vi "TB-Update Spectrum Average.vi"(5 "mic signal":dbl[](array[numeric]), 7 "state in":T1) -> (4 "RMS":dbl, 6 "+Freq. Mag of FFT (dB rms) out":dbl[](array[numeric]), 8 "state out":T1)   [LabVIEW 2020]
uses:
  Typedefs/TB-Runtime state.ctl
  <vilib>/sound2/lvsound2.llb/Sound File Refnum.ctl
  Typedefs/TB-Setup Log.ctl
  <vilib>/Analysis/baseanly.llb/Mean.vi
  <vilib>/Analysis/baseanly.llb/Mean (DBL).vi
  epl-vi-lib/Utility VIs/Math VIs/FFT x(t) to dB,Degrees (1D).vi
  epl-vi-lib/Utility VIs/Math VIs/dB to Linear (1D).vi
  epl-vi-lib/Utility VIs/Math VIs/Linear to dB (scalar).vi
  epl-vi-lib/Utility VIs/Math VIs/Linear to dB (array).vi
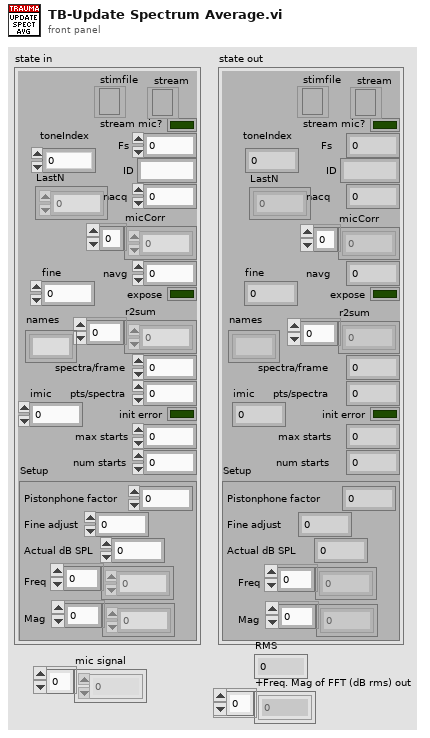
[diagram p1: front panel]
types:
  T1 = typedef "TB-Runtime state.ctl" = cluster{"stimfile":T2, "stream mic?":bool, "Fs":dbl, "ID":string, "micCorr":dbl[], "navg":i32, "r2sum":dbl[], "expose":bool, "spectra/frame":i32, "pts/spectra":i32, "nacq":i32, "init error":bool, "max starts":i32, "num starts":i32, "Setup":T3, "toneIndex":i32, "LastN":dbl[], "fine":dbl, "imic":i32, "stream":refnum<file>, "names":string[]}
  T2 = typedef "Sound File Refnum.ctl" = refnum<file>
  T3 = typedef "TB-Setup Log.ctl" = cluster{"Pistonphone factor":dbl, "Fine adjust":dbl, "Actual dB SPL":dbl, "Freq":dbl[], "Mag":dbl[]}
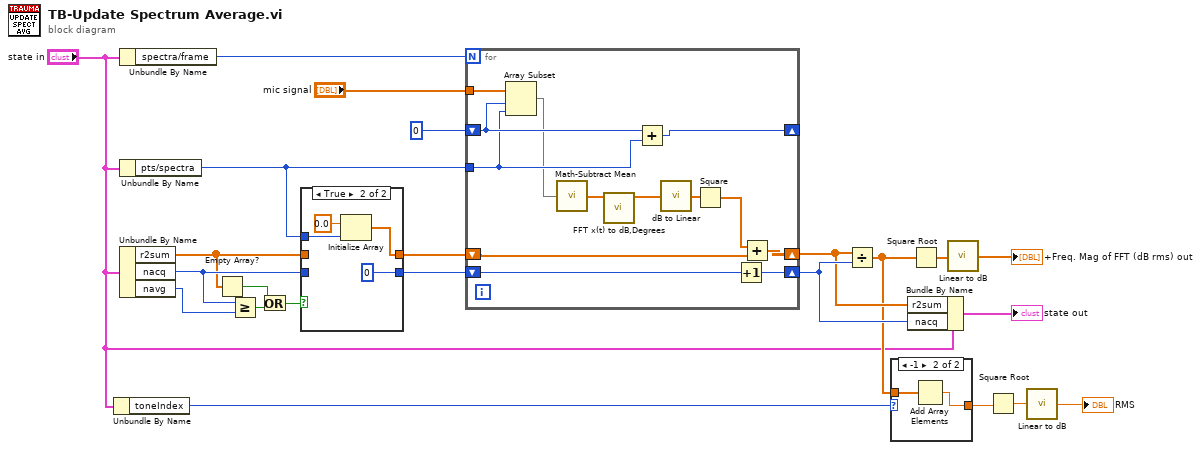
[diagram p0: block diagram]
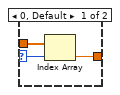
[diagram p3: hidden frame]
diagram:
  n1 = Unbundle By Name("state in") -> ("toneIndex"=w3:i32)
  n2 = Unbundle By Name("state in") -> ("spectra/frame"=w11:i32)
  n3 = Unbundle By Name("state in") -> ("pts/spectra"=w12:i32)
  n4 = Unbundle By Name("state in") -> ("r2sum"=w15:dbl[], "nacq"=w20:i32, "navg"=w10:i32)
  n5 = Empty Array?(array=w15) -> (empty?=w22:bool)
  n6 = Greater Or Equal?(x=w20, y=w10) -> (x >= y?=w23:bool)
  n7 = Or(x=w22, y=w23) -> (x .or. y?=w21:bool)
  n8 = case shown="True" w21 {
    tunnel: w15 -> [w25 _]
    tunnel: [w25 w26] -> w13
    tunnel: w20 -> [w24 _]
    tunnel: [w24 0] -> w14
    tunnel: w12 -> [_ w28]
    frame False {
    }
    frame True {
      n9 = Initialize Array(0.0 ("element"), w28) -> (w26:dbl[])
    }
  }
  n10 = for {
    N: w11 -> [_]
    tunnel: "mic signal" -> [w42]
    shift-right: [w39] -> _
    shift-left: 0 -> [w41]
    tunnel: w12 -> [w40]
    shift-right: [w37] -> w9
    shift-left: w14 -> [w38]
    shift-right: [w35] -> w8
    shift-left: w13 -> [w36]
    n11 = Array Subset(array=w42, index=w41, length=w40) -> (w34:dbl[])
    n12 = call "Math-Subtract Mean.vi"("Y"=w34) -> ("Y - mean(Y)"=w31:dbl[])  [unwired: 4 in]
    n13 = call-poly "FFT x(t) to dB,Degrees.vi"("X"=w31) -> ("+Freq. Mag of FFT (dB rms)"=w30:dbl[])  [unwired: 8 in, 2 out]
    n14 = Add(x=w41, y=w40) -> (x+y=w39:i32)
    n15 = call-poly "dB to Linear.vi"("dB"=w30) -> ("linear"=w33:dbl[])
    n16 = Square(x=w33) -> (x^2=w32:dbl[])
    n17 = Increment(x=w38) -> (x+1=w37:i32)
    n18 = Add(x=w32, y=w36) -> (x+y=w35:dbl[])
  }
  n19 = Divide(x=w8, y=w9) -> (x/y=w4:dbl[])
  n20 = case shown="-1" w3 {
    selector: w3 -> [w45 _]
    tunnel: [w43 w47] -> w1
    tunnel: w4 -> [w44 w46]
    frame 0, Default {
      n21 = Index Array(array=w44, index=w45) -> (element=w43:dbl)
    }
    frame -1 {
      n22 = Add Array Elements(numeric array=w46) -> (sum=w47:dbl)
    }
  }
  n23 = Bundle By Name(cluster="state in", "r2sum"=w8, "nacq"=w9) -> (→"state out":T1)
  n24 = Square Root(x=w4) -> (sqrt(x)=w7:dbl[])
  n25 = call-poly "Linear to dB.vi"("linear"=w7) -> ("dB"=→"+Freq. Mag of FFT (dB rms) out":dbl[])
  n26 = Square Root(x=w1) -> (sqrt(x)=w18:dbl)
  n27 = call-poly "Linear to dB.vi"("Linear"=w18) -> ("dB"=→"RMS":dbl)
